vi "ParseArgumentsCore.vi"(8 "error in (no error)":errorcluster, 10 "Inputs":string[](array[string]), 11 "RunVI in":refnum<class "RunVI.lvclass">) -> (0 "error out":errorcluster, 3 "RunVI out":refnum<class "RunVI.lvclass">)   [LabVIEW 2014, in "RunVI.lvclass"]
uses:
  RunVI.lvclass
  RunVI.lvclass/RunVI.ctl
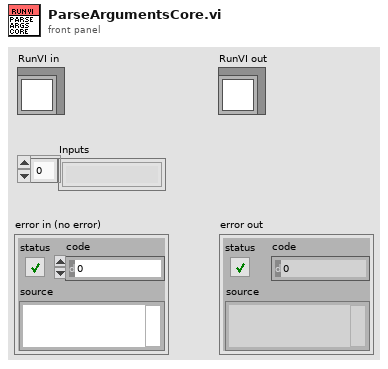
[diagram p1: front panel]
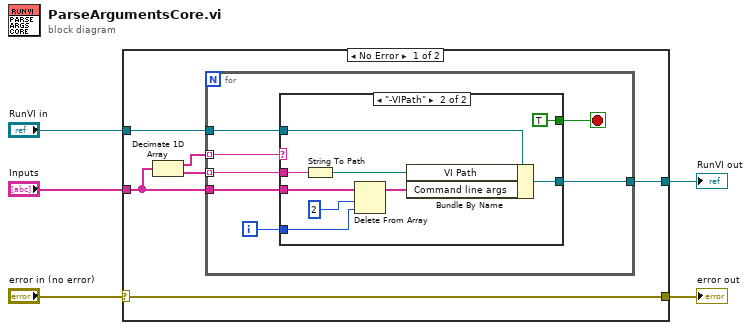
[diagram p0: block diagram]
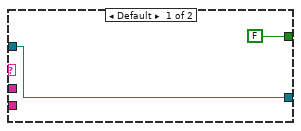
[diagram p2: hidden frame]
diagram:
  n1 = case shown="No Error" "error in (no error)" {
    selector: "error in (no error)" -> [w6 w31]
    tunnel: "Inputs" -> [w11 _]
    tunnel: [w9 w30] -> w4
    tunnel: "RunVI in" -> [w7 w30]
    tunnel: [w6 w31] -> w1
    frame No Error {
      n2 = Decimate 1D Array(w11) -> (w8:string[], w10:string[])
      n3 = for {
        tunnel: w8 -> [w18] mode=indexing
        tunnel: w7 -> [w17]
        tunnel: [w15] -> w9
        tunnel: w10 -> [w14] mode=indexing
        tunnel: w11 -> [w12]
        i -> [w13]
        stop <- w16 stop-if-true
        n4 = case shown="\"-VIPath\"" w18 {
          tunnel: w17 -> [w19 w28]
          tunnel: [FALSE TRUE] -> w16
          tunnel: [w19 w27] -> w15
          tunnel: w14 -> [_ w25]
          tunnel: w13 -> [_ w24]
          tunnel: w12 -> [_ w22]
          frame Default {
          }
          frame "-VIPath" {
            n5 = String To Path(string=w25) -> (path=w26:path)
            n6 = Delete From Array(array=w22, length=2, index=w24) -> (array with subset deleted=w21:string[])  [unwired: 1 out]
            n7 = Bundle By Name(cluster=w28, "VI Path"=w26, "Command line args"=w21) -> (w27:refnum<class "RunVI.lvclass">)
          }
        }
      }
    }
    frame Error {
    }
  }
  "RunVI out" <- w4
  "error out" <- w1
